vi "Obtain Notifiers and Queue.vi"(8 "error in (no error)":errorcluster, 11 "DAQmx":refnum<class "DAQmx.lvclass">) -> (0 "error out":errorcluster, 2 "output cluster":T1, 3 "DAQmx out":refnum<class "DAQmx.lvclass">)   [LabVIEW 2019, in "DAQmx.lvclass"]
uses:
  DAQmx.lvclass
  typedefs/DAQmx.States--enum.ctl
  typedefs/DAQ.Config.AO--Cluster--Array.ctl
  typedefs/DAQ.Config.AO--Cluster.ctl
  typedefs/DAQ.Config.AO.Range--enum.ctl
  typedefs/DAQ.Config.Device Type--enum.ctl
  typedefs/DAQ.Config.AI--Cluster--Array.ctl
  typedefs/DAQ.Config.AI--Cluster.ctl
  typedefs/DAQ.Config.AI.Coupling--enum.ctl
  typedefs/DAQ.Config.AI.Range--enum.ctl
  typedefs/DAQ.Config.Timing--Cluster.ctl
  typedefs/DAQ.Config.Timing.Sampling--Cluster.ctl
  typedefs/DAQ.Config.Timing.Fs Mode--enum.ctl
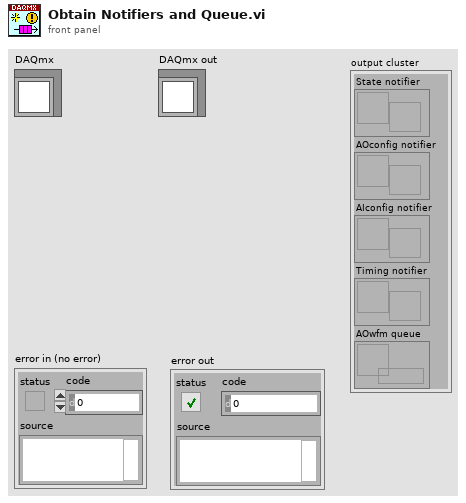
[diagram p1: front panel]
types:
  T1 = cluster{"State notifier":refnum<notifier>, "AOconfig notifier":refnum<notifier>, "AIconfig notifier":refnum<notifier>, "Timing notifier":refnum<notifier>, "AOwfm queue":refnum<queue>}
  T2 = typedef "DAQmx.lvclass/PrivateEvents--Cluster.ctl" = cluster{"State":refnum<user-event>, "AOconfig":refnum<user-event>, "AIconfig":refnum<user-event>, "Timing":refnum<user-event>, "AOwfm":refnum<user-event>}
  T3 = typedef "DAQmx.lvclass/DAQ.Config.Timing--Cluster.ctl" = cluster{"Sampling":T4, "sample mode":i32, "FsMode":T5, "Fs Multiplier":dbl, "Refresh Rate (Hz)":dbl, "Decimation.PreDSP":i32, "Decimation.PostDSP":i32, "Fs.Output":dbl}
  T4 = typedef "DAQmx.lvclass/DAQ.Config.Timing.Sampling--Cluster.ctl" = cluster{"Fs":dbl, "#s":i32}
  T5 = typedef "DAQmx.lvclass/DAQ.Config.Timing.Fs Mode--enum.ctl" = enum16{"Manual", "Auto Fs", "Max Fs"}
  T6 = typedef "DAQmx.lvclass/DAQmx.States--enum.ctl" = enum16{"idle", "start", "stop", "calibrate", "auto"}
  T7 = typedef "DAQmx.lvclass/DAQ.Config.AO--Cluster--Array.ctl" = T8[]
  T8 = typedef "DAQmx.lvclass/DAQ.Config.AO--Cluster.ctl" = cluster{"Channels":tag, "Range":T9, "output terminal configuration":i32, "Type":T10}
  T9 = typedef "DAQmx.lvclass/DAQ.Config.AO.Range--enum.ctl" = enum16{"±0.1", "±1.0", "±10.0", ""}
  T10 = typedef "DAQmx.lvclass/DAQ.Config.Device Type--enum.ctl" = enum16{"None", "USB-4431", "PXI-446x"}
  T11 = typedef "DAQmx.lvclass/DAQ.Config.AI--Cluster--Array.ctl" = T12[]
  T12 = typedef "DAQmx.lvclass/DAQ.Config.AI--Cluster.ctl" = cluster{"Channels":tag, "Coupling":T13, "Range":T14, "input terminal configuration":i32, "Type":T10}
  T13 = typedef "DAQmx.lvclass/DAQ.Config.AI.Coupling--enum.ctl" = u16
  T14 = typedef "DAQmx.lvclass/DAQ.Config.AI.Range--enum.ctl" = enum16{"±0.316", "±1.00", "±3.16", "±10.0", "±31.6", "±42.4", ""}
  T15 = cluster{"setState":T6, "AOconfig":T7, "AIconfig":T11, "Timing":T3, "AOwfm":waveform(dbl)[]}
  T16 = cluster{"notifier out":refnum<notifier>, "notifier out":refnum<notifier>, "notifier out":refnum<notifier>, "notifier out":refnum<notifier>, "queue out":refnum<queue>}
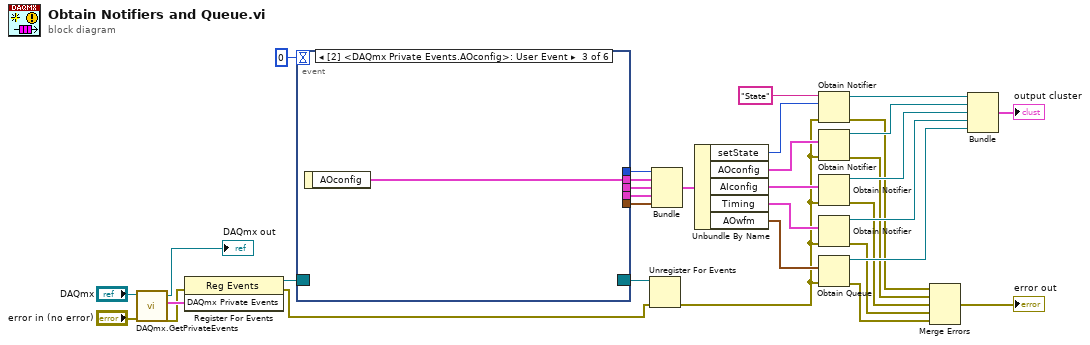
[diagram p0: block diagram]
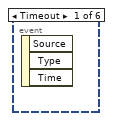
[diagram p2: hidden frame]
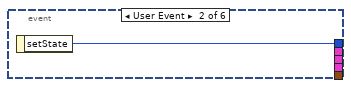
[diagram p3: hidden frame]
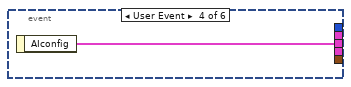
[diagram p4: hidden frame]
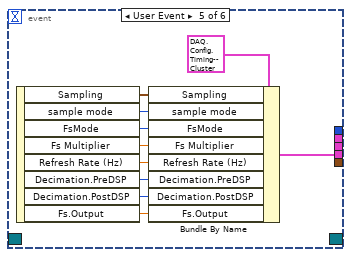
[diagram p5: hidden frame]
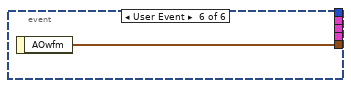
[diagram p6: hidden frame]
diagram:
  n1 = call "DAQmx.GetPrivateEvents.vi"("error in (no error)"="error in (no error)", "DAQmx"="DAQmx") -> ("error out"=w22:errorcluster, "DAQmx Private Events"=w29:T2, "DAQmx out"=→"DAQmx out":refnum<class "DAQmx.lvclass">)  [unwired: 7 in]
  n2 = register-events(error in=w22, w29) -> (reference out=w28:refnum<event-registration>, error out=w24:errorcluster)  [unwired: 1 in]
  n3 = event shown="[2] <DAQmx Private Events.AOconfig>: User Event" {
    selector: w28 -> [_ _ _ _ _ _]
    dyn-events: [_ _ _ _ _ _] -> w25
    timeout: 0 -> [_ _ _ _ _ _]
    tunnel: [_ w35 _ _ _ _] -> w34
    tunnel: [_ _ w36 _ _ _] -> w33
    tunnel: [_ _ _ w37 _ _] -> w32
    tunnel: [_ _ _ _ w46 _] -> w31
    tunnel: [_ _ _ _ _ w48] -> w30
    event Timeout {
      n4 = event-data() -> ()  [unwired: 1 in, 3 out]
    }
    event User Event {
      n5 = event-data() -> ("setState"=w35:T6)  [unwired: 1 in]
    }
    event User Event {
      n6 = event-data() -> ("AOconfig"=w36:T7)  [unwired: 1 in]
    }
    event User Event {
      n7 = event-data() -> ("AIconfig"=w37:T11)  [unwired: 1 in]
    }
    event User Event {
      n8 = event-data() -> ("Sampling"=w45:T4, "sample mode"=w44:i32, "FsMode"=w43:T5, "Fs Multiplier"=w42:dbl, "Refresh Rate (Hz)"=w41:dbl, "Decimation.PreDSP"=w40:i32, "Decimation.PostDSP"=w39:i32, "Fs.Output"=w38:dbl)  [unwired: 1 in]
      n9 = Bundle By Name(cluster=T3 {"Sampling"={"Fs"=1000.0, "#s"=128}, "sample mode"=10123, "FsMode"=enum."Manual", "Fs Multiplier"=1.0, "Refresh Rate (Hz)"=10.0, "Decimation.PreDSP"=1, "Decimation.PostDSP"=1, "Fs.Output"=204789.0} ("Timing"), "Sampling"=w45, "sample mode"=w44, "FsMode"=w43, "Fs Multiplier"=w42, "Refresh Rate (Hz)"=w41, "Decimation.PreDSP"=w40, "Decimation.PostDSP"=w39, "Fs.Output"=w38) -> (w46:T3)
    }
    event User Event {
      n10 = event-data() -> ("AOwfm"=w48:waveform(dbl)[])  [unwired: 1 in]
    }
  }
  n11 = Unregister For Events(event registration refnum=w25, error in=w24) -> (error out=w8:errorcluster)
  n12 = Bundle("setState"=w34, "AOconfig"=w33, "AIconfig"=w32, "Timing"=w31, "AOwfm"=w30) -> (w27:T15)  [unwired: 1 in]
  n13 = Unbundle By Name(w27) -> ("setState"=w21:T6, "AOconfig"=w18:T7, "AIconfig"=w20:T11, "Timing"=w19:T3, "AOwfm"=w9:waveform(dbl)[])
  n14 = Obtain Notifier(name (unnamed)="State", notification data type=w21, error in (no error)=w8) -> (notifier out=w11:refnum<notifier>, error out=w7:errorcluster)  [unwired: 1 in, 1 out]
  n15 = Obtain Notifier(notification data type=w18, error in (no error)=w8) -> (notifier out=w17:refnum<notifier>, error out=w6:errorcluster)  [unwired: 2 in, 1 out]
  n16 = Obtain Notifier(notification data type=w20, error in (no error)=w8) -> (notifier out=w16:refnum<notifier>, error out=w5:errorcluster)  [unwired: 2 in, 1 out]
  n17 = Obtain Notifier(notification data type=w19, error in (no error)=w8) -> (notifier out=w14:refnum<notifier>, error out=w4:errorcluster)  [unwired: 2 in, 1 out]
  n18 = Obtain Queue(element data type=w9, error in (no error)=w8) -> (queue out=w15:refnum<queue>, error out=w3:errorcluster)  [unwired: 3 in, 1 out]
  n19 = Merge Errors(w7, w6, w5, w4, w3) -> (→"error out":errorcluster)
  n20 = Bundle("notifier out"=w11, "notifier out"=w17, "notifier out"=w16, "notifier out"=w14, "queue out"=w15) -> (→"output cluster":T16)  [unwired: 1 in]
